vi "cont_array.vi"(7 "ignore_first_edge?":bool, 8 "edge cluster":cluster{"Array":i16[], "Array":bool[]}, 11 "u8_ar_phase map":u8[](array[numeric])) -> (3 "Array":i16[](array[numeric]))   [LabVIEW 2011]
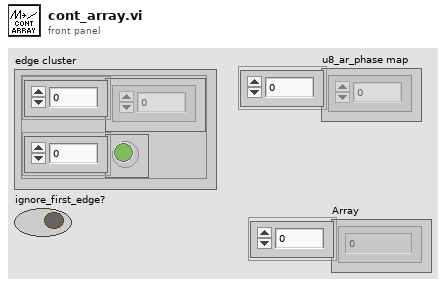
[diagram p1: front panel]
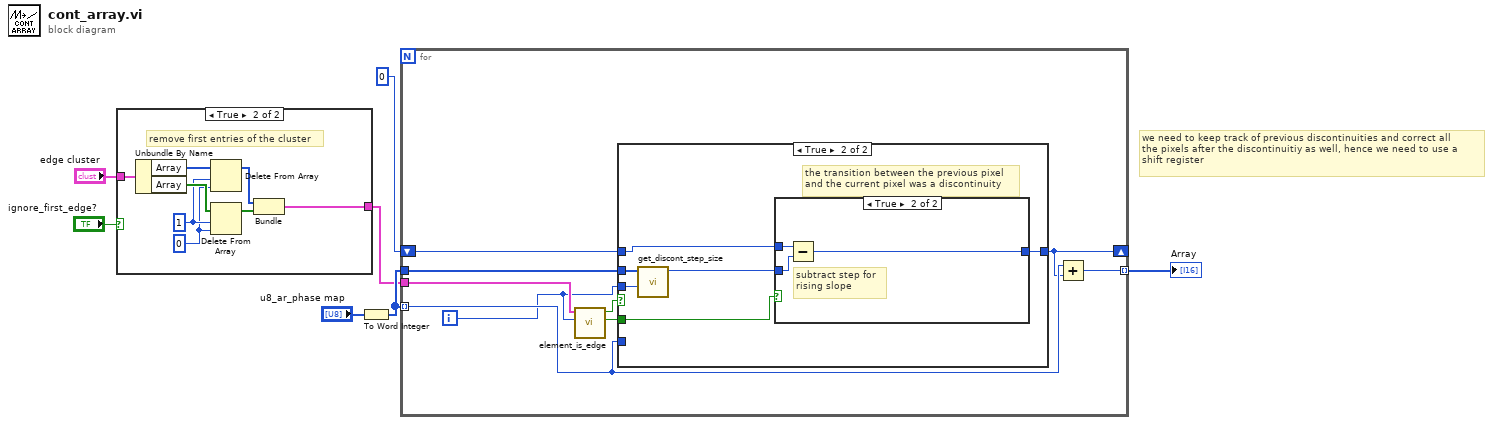
[diagram p0: block diagram]
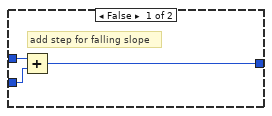
[diagram p4: hidden frame]
diagram:
  # "we need to keep track of previous discontinuities and correct all \nthe pixels after the discontinuitiy as well, hence we need to use a \nshift register"
  n1 = case shown="True" "ignore_first_edge?" {
    tunnel: "edge cluster" -> [w8 w10]
    tunnel: [w8 w9] -> w2
    frame False {
    }
    frame True {
      w14 = 1 ("length")
      w13 = 0 ("index")
      # "remove first entries of the cluster"
      n2 = Unbundle By Name(w10) -> ("Array"=w16:i16[], "Array"=w15:bool[])
      n3 = Delete From Array(array=w16, length=w14, index=w13) -> (array with subset deleted=w12:i16[])  [unwired: 1 out]
      n4 = Delete From Array(array=w15, length=w14, index=w13) -> (array with subset deleted=w11:bool[])  [unwired: 1 out]
      n5 = Bundle("Array"=w12, "Array"=w11) -> (w9:cluster{"Array":i16[], "Array":bool[]})  [unwired: 1 in]
    }
  }
  n6 = To Word Integer(number="u8_ar_phase map") -> (16bit integer=w5:i16[])
  n7 = for {
    tunnel: w5 -> [w21]
    tunnel: w5 -> [w23] mode=indexing
    shift-right: [w20] -> _
    shift-left: i16 0 -> [w25]
    tunnel: [w24] -> w4 mode=indexing
    tunnel: w2 -> [w22]
    i -> [w19]
    n8 = call "element_is_edge.vi"("current element"=w19, "edge cluster"=w22) -> ("direction (rising/falling)"=w17:bool, "edge"=w18:bool)  [unwired: 8 in]
    n9 = case shown="True" w18 {
      tunnel: [w26 w31] -> w20
      tunnel: w25 -> [w26 w32]
      tunnel: w17 -> [_ w30]
      tunnel: w23 -> [_ _]
      tunnel: w19 -> [_ w28]
      tunnel: w21 -> [_ w29]
      frame False {
      }
      frame True {
        # "the transition between the previous pixel\nand the current pixel was a discontinuity"
        n10 = call "get_discont_step_size.vi"("current pixel (iteration)"=w28, "current row in image"=w29) -> ("step_size"=w27:i16)  [unwired: 9 in]
        n11 = case shown="True" w30 {
          tunnel: w32 -> [w35 w38]
          tunnel: [w34 w37] -> w31
          tunnel: w27 -> [w33 w36]
          frame False {
            # "add step for falling slope"
            n12 = Add(x=w35, y=w33) -> (x+y=w34:i16)
          }
          frame True {
            # "subtract step for \nrising slope"
            n13 = Subtract(x=w38, y=w36) -> (x-y=w37:i16)
          }
        }
      }
    }
    n14 = Add(x=w23, y=w20) -> (x+y=w24:i16)
  }
  "Array" <- w4
